vi "EJERCICIO 2.vi"() -> ()   [LabVIEW 2014]
panel:
  out "EL NUMERO ES:":string
  out "Boolean":bool
  in  "INGRESE EL NUMERO":dbl
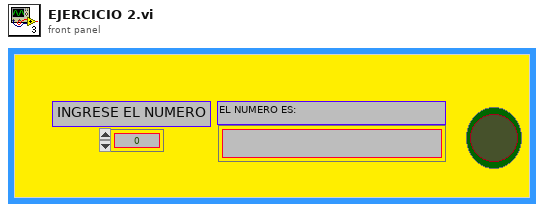
[diagram p1: front panel]
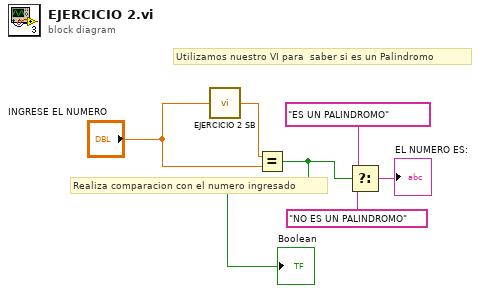
[diagram p0: block diagram]
diagram:
  # "Realiza comparacion con el numero ingresado"
  # "Utilizamos nuestro VI para  saber si es un Palindromo"
  n1 = call "EJERCICIO 2 SB.vi"("INGRESE UN NUMERO"="INGRESE EL NUMERO") -> ("NUMERO INVERTIDO"=w2:dbl)
  n2 = Equal?(x=w2, y="INGRESE EL NUMERO") -> (x = y?=w4:bool)
  "Boolean" <- w4
  n3 = Select(t="ES UN PALINDROMO", s=w4, f="NO ES UN PALINDROMO") -> (s? t:f=→"EL NUMERO ES:":string)
